vi "RFWindow.vi"(4 "rf points per line":i32, 5 "Sample Time":dbl format="%.2e", 6 "Sampling (Hz) In":dbl, 7 "Text of Samp Rate":string) -> (1 "curser position":dbl format="%.2f", 3 "Sampling (Hz)":dbl)   [LabVIEW 2022 SP3]
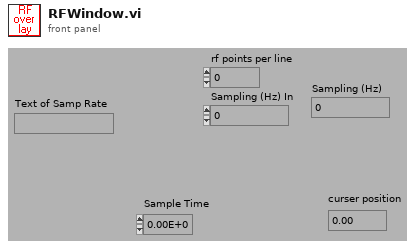
[diagram p1: front panel]
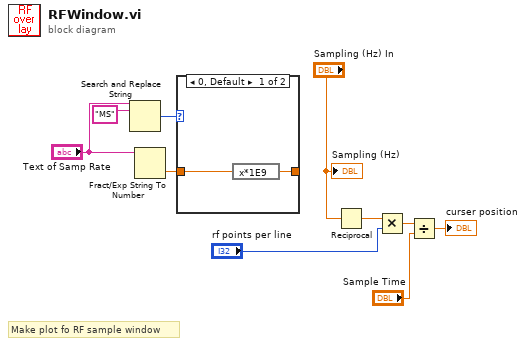
[diagram p0: block diagram]
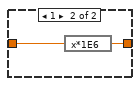
[diagram p2: hidden frame]
diagram:
  # "Make plot fo RF sample window"
  n1 = Search and Replace String(input string="Text of Samp Rate", search string="MS") -> (number of replacements=w5:i32)  [unwired: 1 in, 8 out]
  n2 = Fract/Exp String To Number(string="Text of Samp Rate") -> (number=w4:dbl)  [unwired: 4 out]
  n3 = case shown="0, Default" w5 {
    tunnel: w4 -> [w12 w14]
    tunnel: [w11 w13] -> _
    frame 0, Default {
      n4 = expression code="x*1E9"(w12) -> (w11:dbl)
    }
    frame 1 {
      n5 = expression code="x*1E6"(w14) -> (w13:dbl)
    }
  }
  n6 = Reciprocal(x="Sampling (Hz) In") -> (1/x=w3:dbl)
  n7 = Multiply(x=w3, y="rf points per line") -> (x*y=w7:dbl)
  n8 = Divide(x=w7, y="Sample Time") -> (x/y=→"curser position":dbl)
  "Sampling (Hz)" <- "Sampling (Hz) In"
